vi "Exercise 7.1.vi"() -> ()   [LabVIEW 2020]
panel:
  out "Walk Sign":bool
  out "Green":bool
  out "Yellow":bool
  out "Red":bool
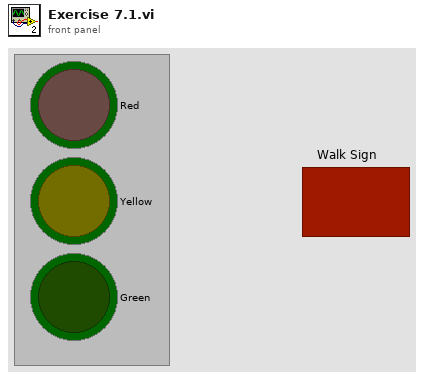
[diagram p1: front panel]
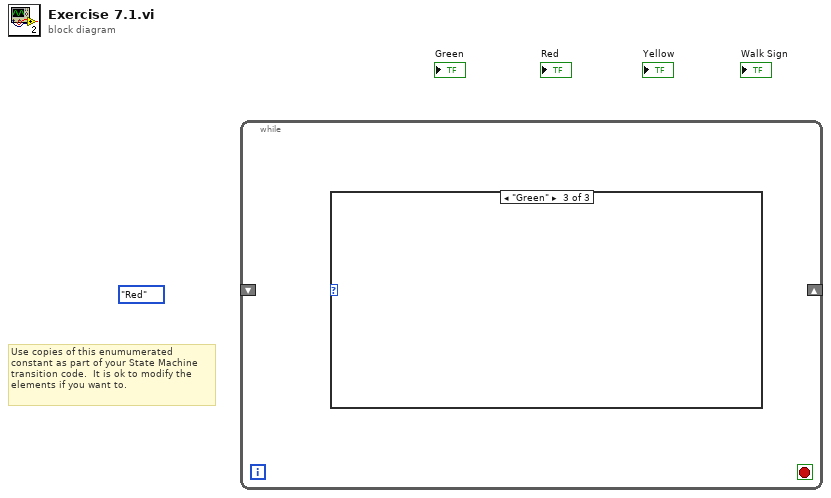
[diagram p0: block diagram]
diagram:
  (unwired) enum16{"Green", "Yellow", "Red"}."Red"
  # "Use copies of this enumumerated \nconstant as part of your State Machine\ntransition code.  It is ok to modify the\nelements if you want to."
  n1 = while {
    shift-right: _ -> [_]
    shift-left: _ -> [_]
    stop <- _ stop-if-true
    n2 = case shown="\"Green\"" {
      selector: _ -> [_ _ _]
      frame "Red", Default {
      }
      frame "Yellow" {
      }
      frame "Green" {
      }
    }
  }
